vi "Previous Album.vi"(8 "Error In":errorcluster, 9 "Current Album":i32, 10 "AlbumArray":T2, 11 "UI Refs":T1) -> (0 "Error Out":errorcluster, 1 "Current Album":i32, 3 "Album Index":string)   [LabVIEW 2015]
uses:
  Controls & Type Defs/UI Data.ctl
  Controls & Type Defs/AlbumArray.ctl
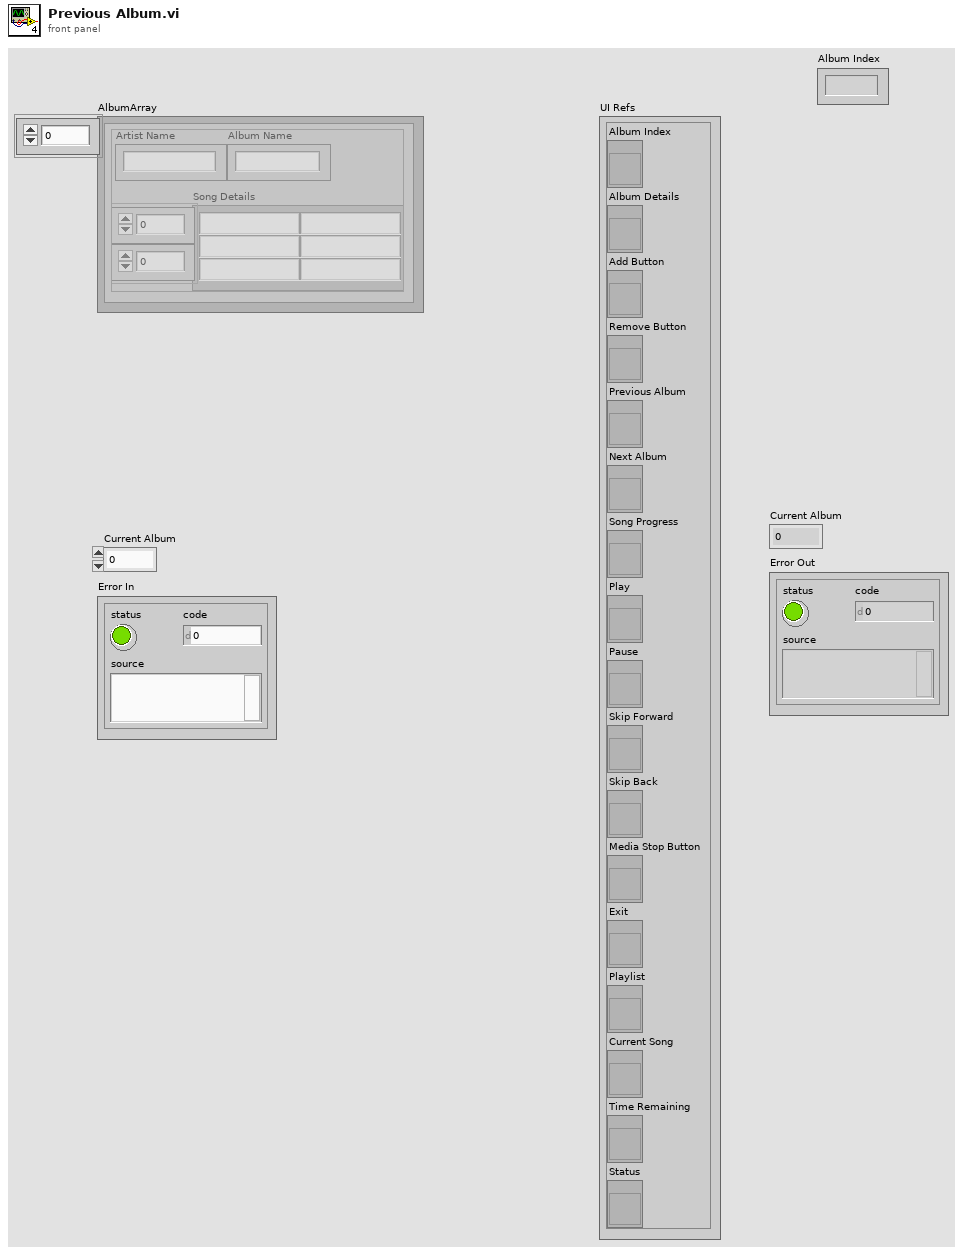
[diagram p1: front panel]
types:
  T1 = typedef "UI Data.ctl" = cluster{"Album Index":refnum<vi>, "Album Details":refnum<vi>, "Add Button":refnum<vi>, "Remove Button":refnum<vi>, "Previous Album":refnum<vi>, "Next Album":refnum<vi>, "Song Progress":refnum<vi>, "Play":refnum<vi>, "Pause ":refnum<vi>, "Skip Forward":refnum<vi>, "Skip Back":refnum<vi>, "Media Stop Button":refnum<vi>, "Exit":refnum<vi>, "Playlist":refnum<vi>, "Current Song":refnum<vi>, "Time Remaining":refnum<vi>, "Status":refnum<vi>}
  T2 = typedef "AlbumArray.ctl" = cluster{"Artist Name":string, "Album Name":string, "Song Details":string[][]}[]
  T3 = cluster{"Artist Name":string, "Album Name":string, "Song Details":string[][]}
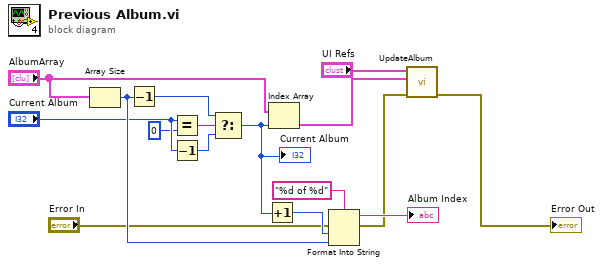
[diagram p0: block diagram]
diagram:
  n1 = Array Size(array="AlbumArray") -> (size(s)=w14:i32)
  n2 = Decrement(x=w14) -> (x-1=w5:i32)
  n3 = Equal?(x="Current Album", y=0 ("t")) -> (x = y?=w8:bool)
  n4 = Decrement(x="Current Album") -> (x-1=w10:i32)
  n5 = Select(t=w5, s=w8, f=w10) -> (s? t:f=w12:i32)
  "Current Album" <- w12
  n6 = Increment(x=w12) -> (x+1=w13:i32)
  n7 = Index Array(array="AlbumArray", index=w12) -> (element=w3:T3)
  n8 = Format Into String(format string="%d of %d", error in="Error In", w13, w14) -> (resulting string=→"Album Index":string, error out=w2:errorcluster)  [unwired: 1 in]
  n9 = call "UpdateAlbum.vi"("error in"=w2, "AlbumArray"=w3, "UI Refs"="UI Refs") -> ("error out"=→"Error Out":errorcluster)  [unwired: 7 in, 1 out]
